vi "Blockchain example.vi"() -> ()   [LabVIEW 2013]
uses:
  JSONtext.lvlib
  <vilib>/gmath/NI_Gmath.lvlib
  <vilib>/addons/JSON API/Get Polymorphic/JSON GetSet.lvlib
  <vilib>/addons/JSON API/Variant JSON/Get as Variant.vi
  <vilib>/addons/JSON API/Variant JSON/Variant JSON.lvlib
  <vilib>/addons/JSON API/JSON Value/Set from JSON string.vi
  <vilib>/addons/JSON API/JSON Value/JSON Value.lvclass
panel:
  out "<JSON>out":string[](array[string])
  out "<JSON>inputs":string[](array[string])
  out "inputs":T1(array[cluster])
  out "out":T2(array[cluster])
  out "Array":dbl[](array[numeric])=[1.23456, 1.23456, 1.23456, 1.23456, 1.23456, 1.23456, 1.23456, 1.23456, 1.23456, 1.23456, 1.23456, 1.23456, 2.23456]
  out "Blockchain 2":T3
  out "Missing":string
  out "Blockchain":T4
  in  "Old JSON":enum16{"JSONtext", "NI", "Old"}(ring)
  out "mean":dbl format="%.3p"
  out "length":i32
  out "Variant out":variant
  out "To Variant":dbl[](array[numeric]) format="%#_3p"
  in  "<JSON>":string="{\n    \"op\": \"utx\",\n    \"x\": {\n        \"lock_time\": 0,\n        \"ver\": 1,\n        \"size\": 192,\n        \"inputs\": [\n            {\n                \"sequence\": 4294967295,\n                \"prev_out\": {\n                    \"spent\": true,\n                    \"tx_index\": 99005468,\n                    \"type\": 0,\n                    \"addr\": \"1BwGf3z7n2fHk6NoVJNkV32qwyAYsMhkWf\",\n                    \"value\": 65574000,\n                    \"n\": 0,\n                    \"script\": \"76a91477f4c9ee75e449a74c21a4decfb50519cbc245b388ac\"\n                },\n                \"script\": \"483045022100e4ff962c292705f051c2c2fc519fa775a4d8955bce1a3e29884b2785277999ed02200b537ebd22a9f25fbbbcc9113c69c1389400703ef2017d80959ef0f1d685756c012102618e08e0c8fd4c5fe539184a30fe35a2f5fccf7ad62054cad29360d871f8187d\"\n            }\n        ],\n        \"time\": 1440086763,\n        \"tx_index\": 99006637,\n        \"vin_sz\": 1,\n        \"hash\": \"0857b9de1884eec314ecf67c040a2657b8e083e1f95e31d0b5ba3d328841fc7f\",\n        \"vout_sz\": 1,\n        \"relayed_by\": \"127.0.0.1\",\n        \"out\": [\n            {\n                \"spent\": false,\n                \"tx_index\": 99006637,\n                \"type\": 0,\n                \"addr\": \"1A828tTnkVFJfSvLCqF42ohZ51ksS3jJgX\",\n                \"value\": 65564000,\n                \"n\": 0,\n                \"script\": \"76a914640cfdf7b79d94d1c980133e3587bd6053f091f388ac\"\n            }\n        ]\n    }\n}"
  out "error out":errorcluster
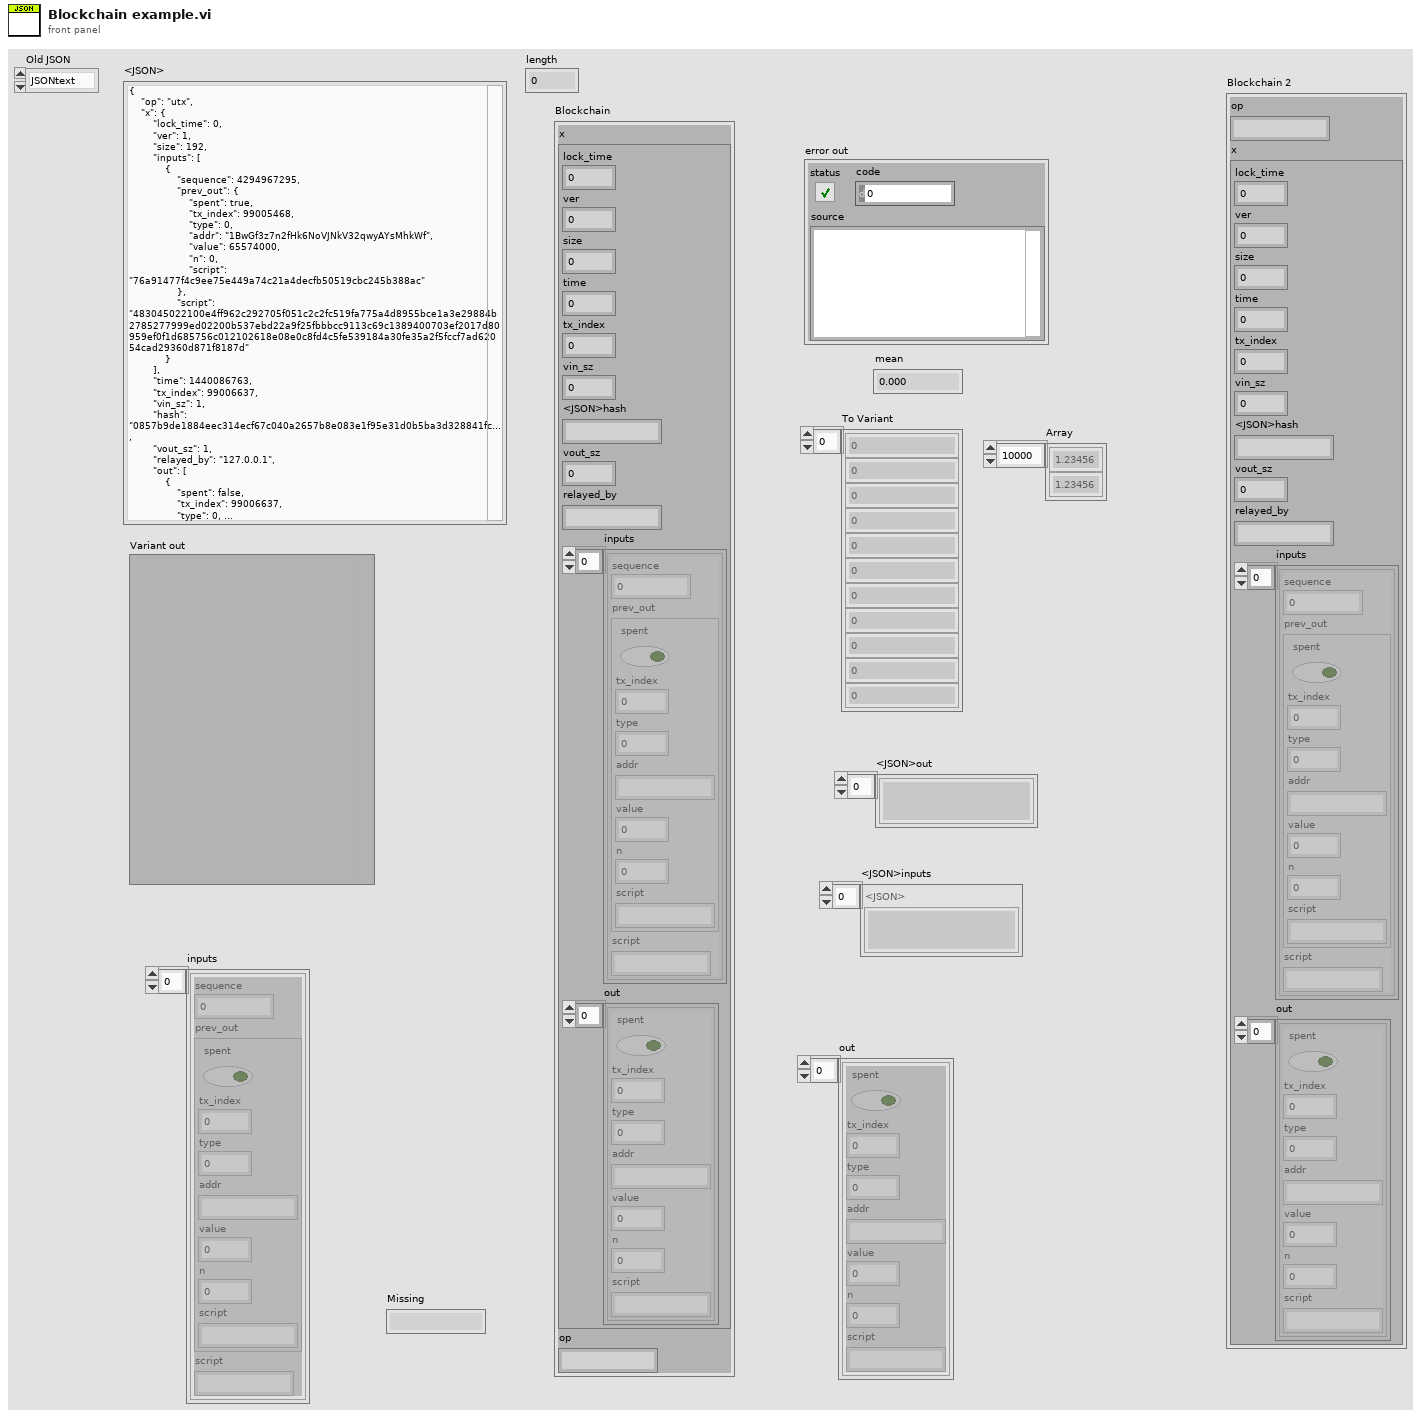
[diagram p1: front panel]
types:
  T1 = cluster{"sequence":i64, "prev_out":cluster{"spent":bool, "tx_index":i32, "type":i32, "addr":string, "value":i32, "n":i32, "script":string}, "script":string}[]
  T2 = cluster{"spent":bool, "tx_index":i32, "type":i32, "addr":string, "value":i32, "n":i32, "script":string}[]
  T3 = cluster{"op":string, "x":cluster{"lock_time":i32, "ver":i32, "size":i32, "time":i32, "tx_index":i32, "vin_sz":i32, "<JSON>hash":string, "vout_sz":i32, "relayed_by":string, "inputs":cluster{"sequence":i64, "prev_out":cluster{"spent":bool, "tx_index":i32, "type":i32, "addr":string, "value":i32, "n":i32, "script":string}, "script":string}[], "out":cluster{"spent":bool, "tx_index":i32, "type":i32, "addr":string, "value":i32, "n":i32, "script":string}[]}}
  T4 = cluster{"x":cluster{"lock_time":i32, "ver":i32, "size":i32, "time":i32, "tx_index":i32, "vin_sz":i32, "<JSON>hash":string, "vout_sz":i32, "relayed_by":string, "inputs":cluster{"sequence":i64, "prev_out":cluster{"spent":bool, "tx_index":i32, "type":i32, "addr":string, "value":i32, "n":i32, "script":string}, "script":string}[], "out":cluster{"spent":bool, "tx_index":i32, "type":i32, "addr":string, "value":i32, "n":i32, "script":string}[]}, "op":string}
  T5 = enum16{"arithmetic", "geometric", "harmonic", "trimmed", "median"}
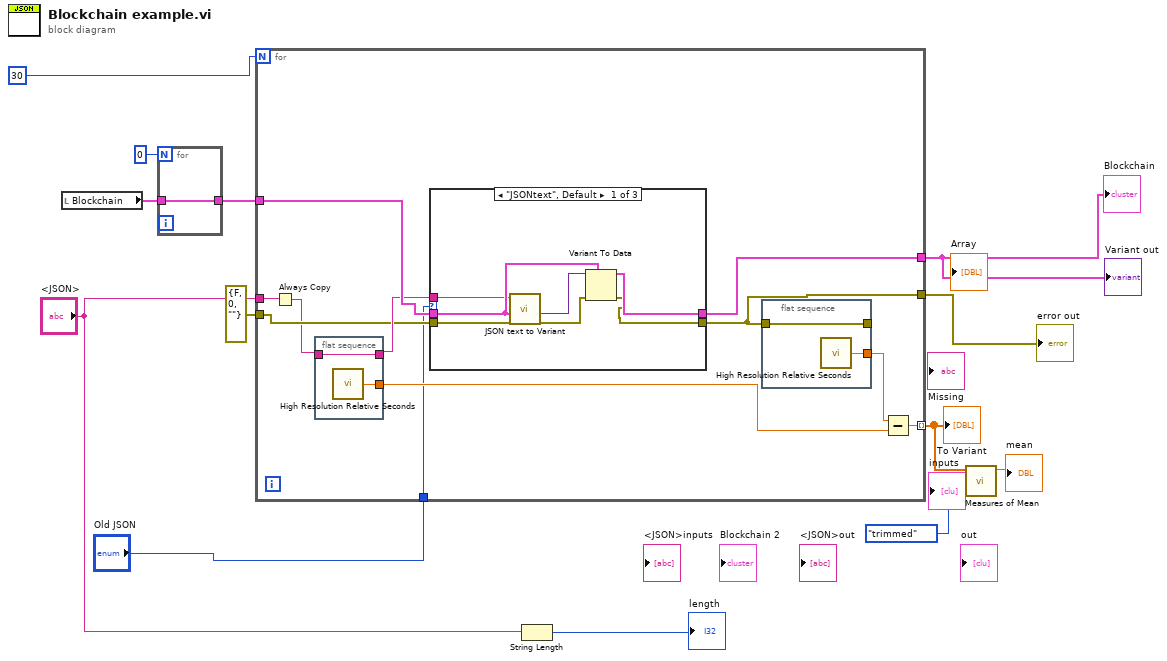
[diagram p0: block diagram]
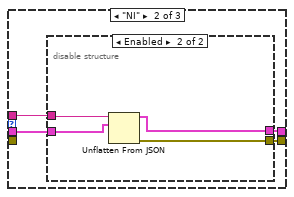
[diagram p2: hidden frame]
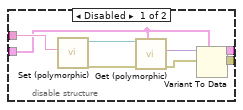
[diagram p3: hidden frame]
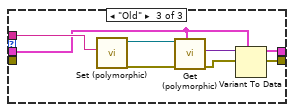
[diagram p4: hidden frame]
diagram:
  n1 = local read "Blockchain"() -> (w11:T4)
  n2 = for {
    N: 0 -> [_]
    tunnel: [w14] -> w12
    tunnel: w11 -> [w14]
  }
  n3 = for {
    N: 30 -> [_]
    tunnel: [w25] -> w6 mode=indexing
    tunnel: w12 -> [w24]
    tunnel: "<JSON>" -> [w20]
    tunnel: [w23] -> w1
    tunnel: errorcluster {"status"=FALSE, "code"=0, "source"=""} ("error out") -> [w18]
    tunnel: "Old JSON" -> [w16]
    tunnel: [w15] -> w2
    n4 = Always Copy(1:w20) -> (0:w17:string)
    n5 = flat-sequence {
      tunnel: [w56] -> w19
      tunnel: w17 -> [w56]
      tunnel: [w55] -> w21
      frame #0 {
        n6 = call <vilib>:"High Resolution Relative Seconds.vi"() -> ("relative seconds"=w55:dbl)
      }
    }
    n7 = case shown="\"JSONtext\", Default" w16 {
      tunnel: w24 -> [w29 w33 w51]
      tunnel: [w30 w34 w52] -> w23
      tunnel: [w27 w35 w53] -> w15
      tunnel: w19 -> [w26 w36 w54]
      tunnel: w18 -> [w32 _ _]
      frame "JSONtext", Default {
        n8 = call "JSON text to Variant.vi"("error in (no error)"=w32, "Variant (Data Type)"=w29, "JSON"=w26) -> ("error out"=w28:errorcluster, "Variant out"=w31:variant)  [unwired: 7 in]
        n9 = Variant To Data(error in=w28, type=w29, Variant=w31) -> (data=w30:T4, error out=w27:errorcluster)
      }
      frame "NI" {
        n10 = disable-structure shown="Enabled" {
          disable-tunnel: w36 -> [w43 w47]
          disable-tunnel: [w40 w44] -> w35
          disable-tunnel: [w38 w45] -> w34
          disable-tunnel: w33 -> [w37 w46]
          frame Disabled {
            n11 = call-poly <vilib>:"Set (polymorphic).vi"("JSON stream"=w43) -> ("error out"=w39:errorcluster, "JSON Value out"=w42:refnum<class "JSON Value.lvclass">)  [unwired: 8 in, 1 out]
            n12 = call-poly <vilib>:"Get (polymorphic).vi"("Variant (Data Type)"=w37, "error in (no error)"=w39, "JSON in"=w42) -> ("error out"=w40:errorcluster, "Variant out"=w41:variant)  [unwired: 6 in, 1 out]
            n13 = Variant To Data(type=w37, Variant=w41) -> (data=w38:T4)  [unwired: 1 in, 1 out]
          }
          frame Enabled {
            n14 = Unflatten From JSON(JSON string=w47, type and defaults=w46) -> (value=w45:T4, error out=w44:errorcluster)  [unwired: 5 in]
          }
        }
      }
      frame "Old" {
        n15 = call-poly <vilib>:"Set (polymorphic).vi"("JSON stream"=w54) -> ("error out"=w48:errorcluster, "JSON Value out"=w50:refnum<class "JSON Value.lvclass">)  [unwired: 8 in, 1 out]
        n16 = call-poly <vilib>:"Get (polymorphic).vi"("Variant (Data Type)"=w51, "error in (no error)"=w48, "JSON in"=w50) -> ("error out"=w53:errorcluster, "Variant out"=w49:variant)  [unwired: 6 in, 1 out]
        n17 = Variant To Data(type=w51, Variant=w49) -> (data=w52:T4)  [unwired: 1 in, 1 out]
      }
    }
    n18 = flat-sequence {
      tunnel: [w58] -> _
      tunnel: w15 -> [w58]
      tunnel: [w57] -> w22
      frame #0 {
        n19 = call <vilib>:"High Resolution Relative Seconds.vi"() -> ("relative seconds"=w57:dbl)
      }
    }
    n20 = Subtract(x=w22, y=w21) -> (x-y=w25:dbl)
  }
  "To Variant" <- w6
  "Variant out" <- w1
  "Blockchain" <- w1
  "error out" <- w2
  n21 = String Length(string="<JSON>") -> (length=→"length":i32)
  n22 = call <vilib>:"Measures of Mean.vi"("type"=T5."trimmed", "x array"=w6) -> ("mean value"=→"mean":dbl)  [unwired: 8 in, 1 out]
